vi "Read Gesture.vi"(8 "error in (no error)":errorcluster, 11 "Grove Gesture Sensor PAJ7620U2 in":refnum<class "Grove Gesture Sensor PAJ7620U2.lvclass">) -> (0 "error out":errorcluster, 2 "Gesture":T1, 3 "Grove Gesture Sensor PAJ7620U2 out":refnum<class "Grove Gesture Sensor PAJ7620U2.lvclass">)   [LabVIEW 2020, in "CTI-Peripheral.lvlib" / "Grove Gesture Sensor PAJ7620U2.lvclass"]
uses:
  Grove Gesture Sensor PAJ7620U2.lvclass
  Base/Gesture.ctl
  Base/Gesture Sensor.lvclass
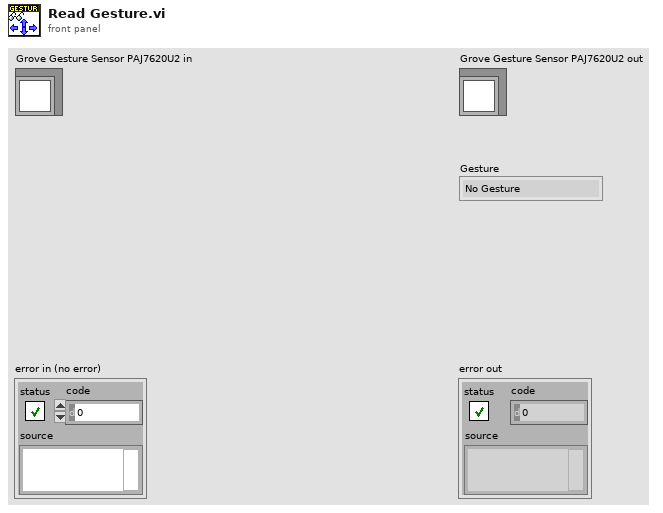
[diagram p1: front panel]
types:
  T1 = typedef "CTI-Peripheral.lvlib/Gesture Sensor.lvclass/Gesture.ctl" = enum16{"No Gesture", "Up", "Down", "Left", "Right", "Forward", "Backward", "Clockwise", "Counterclockwise"}
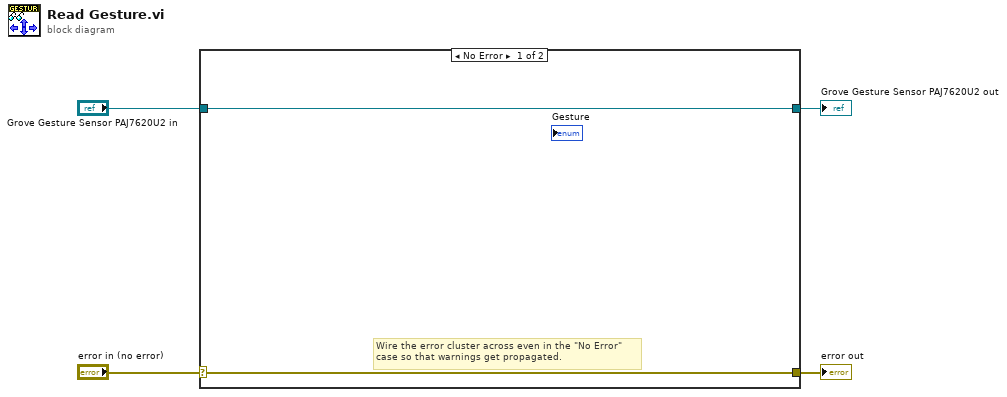
[diagram p0: block diagram]
diagram:
  n1 = case shown="No Error" "error in (no error)" {
    selector: "error in (no error)" -> [w5 w8]
    tunnel: [w5 w8] -> w3
    tunnel: [w6 w7] -> w1
    tunnel: "Grove Gesture Sensor PAJ7620U2 in" -> [w6 w7]
    frame No Error {
      # "Wire the error cluster across even in the \"No Error\"\ncase so that warnings get propagated."
    }
    frame Error {
    }
  }
  "error out" <- w3
  "Grove Gesture Sensor PAJ7620U2 out" <- w1
